vi "SendCommand.vi"(6 "HighPrio":bool, 8 "ErrorIn":errorcluster, 9 "Name":string, 10 "CmdCtrl":T1, 11 "QueueIn":refnum<queue>) -> (0 "ErrorOut":errorcluster)   [LabVIEW 2021, in "YActor.lvclass"]
uses:
  YActor.lvclass
  CmdCtrl.ctl
  AsyncErrorHandling.ctl
  CallMode.ctl
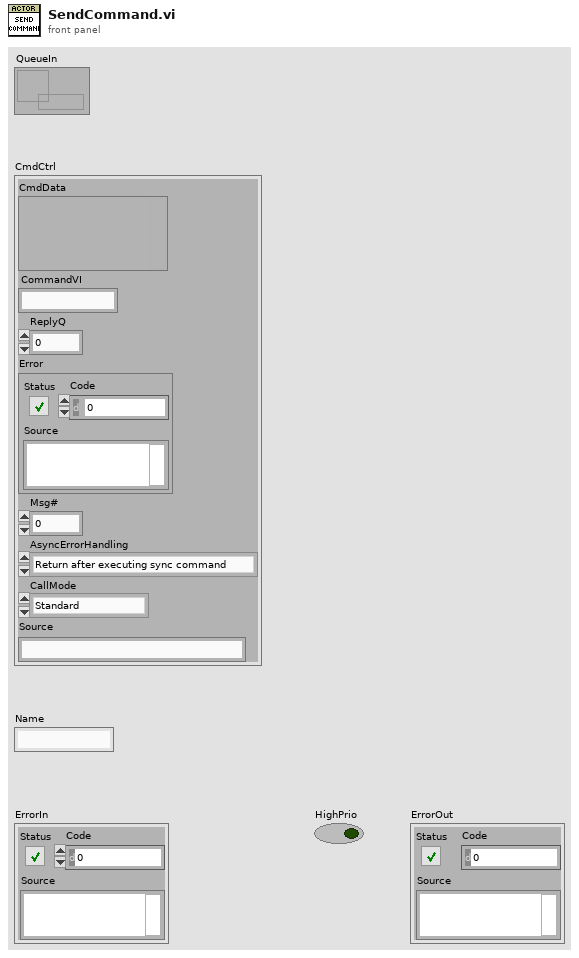
[diagram p1: front panel]
types:
  T1 = typedef "YActor.lvclass/CmdCtrl.ctl" = cluster{"CmdData":variant, "CommandVI":string, "ReplyQ":i64, "Error":errorcluster, "Msg#":u32, "AsyncErrorHandling":T2, "CallMode":T3, "Source":string}
  T2 = typedef "YActor.lvclass/AsyncErrorHandling.ctl" = enum16{"Return after executing sync command", "Return before executing sync command", "Don't return error"}
  T3 = typedef "YActor.lvclass/CallMode.ctl" = enum16{"Standard", "Call&Collect"}
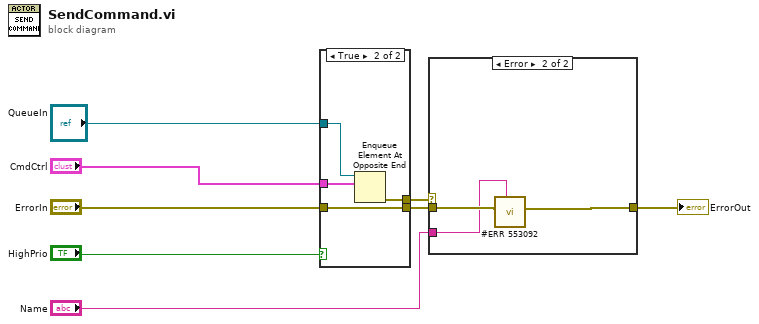
[diagram p0: block diagram]
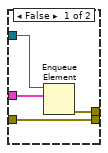
[diagram p3: hidden frame]
diagram:
  n1 = case shown="True" "HighPrio" {
    tunnel: "QueueIn" -> [w10 w14]
    tunnel: "CmdCtrl" -> [w9 w13]
    tunnel: [w12 w16] -> w6
    tunnel: "ErrorIn" -> [w11 w15]
    tunnel: [w11 w15] -> w7
    frame False {
      n2 = Enqueue Element(queue=w10, element=w9) -> (error out=w12:errorcluster)  [unwired: 2 in, 2 out]
    }
    frame True {
      n3 = Enqueue Element At Opposite End(queue=w14, element=w13) -> (error out=w16:errorcluster)  [unwired: 2 in, 2 out]
    }
  }
  n4 = case shown="Error" w6 {
    tunnel: w7 -> [w17 w20]
    tunnel: [w17 w19] -> w8
    tunnel: "Name" -> [_ w18]
    frame No Error {
    }
    frame Error {
      n5 = call "#ERR 553092"("Data"=w18, "error in (no error)"=w20) -> ("error out"=w19:errorcluster)  [unwired: 9 in]
    }
  }
  "ErrorOut" <- w8
